vi "Write ctl.vi"(8 "error in (no error)":errorcluster, 10 "ctl":cluster{"P":dbl, "I":dbl, "D":dbl}, 11 "Update TE Tech PID in":refnum<class "Update TEC PID.lvclass">) -> (0 "error out":errorcluster, 3 "Update TE Tech PID out":refnum<class "Update TEC PID.lvclass">)   [LabVIEW 2014, in "Controller.lvlib" / "Update TEC PID.lvclass"]
uses:
  Update TEC PID.lvclass
  Update TEC PID.lvclass/Update TEC PID.ctl
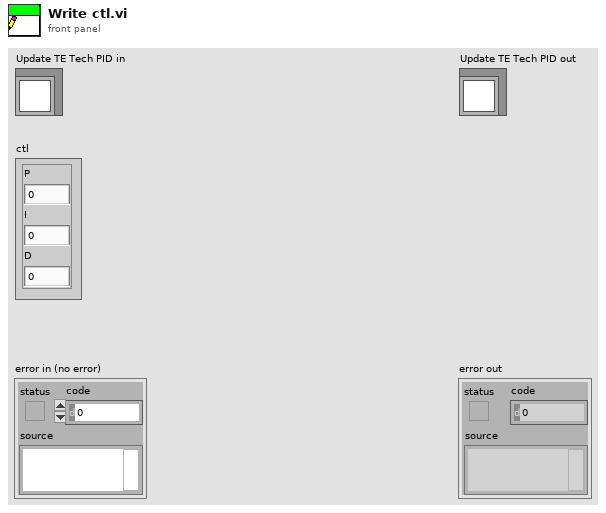
[diagram p1: front panel]
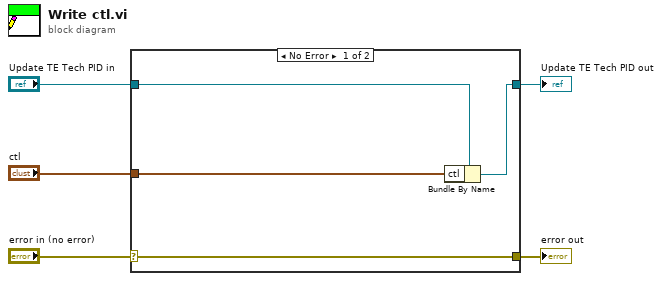
[diagram p0: block diagram]
diagram:
  n1 = case shown="No Error" "error in (no error)" {
    selector: "error in (no error)" -> [w9 w10]
    tunnel: [w9 w10] -> w4
    tunnel: [w7 w11] -> w2
    tunnel: "Update TE Tech PID in" -> [w8 w11]
    tunnel: "ctl" -> [w6 _]
    frame No Error {
      n2 = Bundle By Name(cluster=w8, "ctl"=w6) -> (w7:refnum<class "Update TEC PID.lvclass">)
    }
    frame Error {
    }
  }
  "error out" <- w4
  "Update TE Tech PID out" <- w2
